vi "GetText.vi"(8 "error in":errorcluster, 11 "EngineTags in":refnum<class "EngineTags.lvclass">) -> (0 "error out":errorcluster, 1 "additional text":string, 2 "text":string, 3 "EngineTags out":refnum<class "EngineTags.lvclass">, 4 "glyph":string)   [LabVIEW 2013, in "PL Framework Configuration Tool.lvlib" / "EngineTags.lvclass"]
uses:
  EngineTags.lvclass
  subVIs/Glyphs Status.ctl
  PL Framework Configuration Tool.lvlib
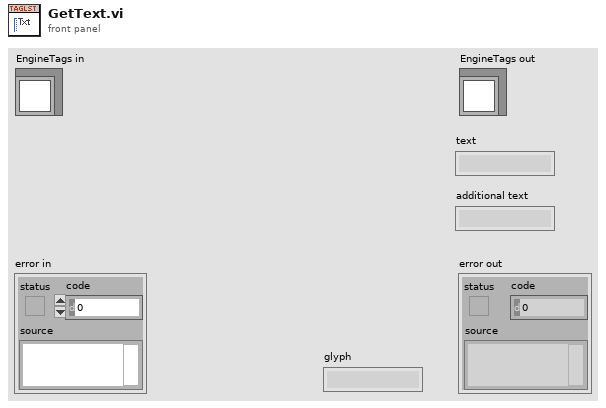
[diagram p1: front panel]
types:
  T1 = typedef "PL Framework Configuration Tool.lvlib/Glyphs Status.ctl" = enum16{"Normal", "Error", "Async"}
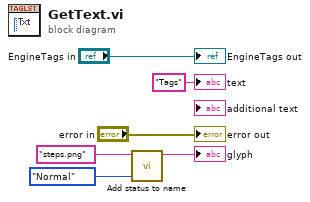
[diagram p0: block diagram]
diagram:
  n1 = call "Add status to name.vi"("Status"=Glyphs_Status."Normal", "Name"="steps.png" ("glyph")) -> ("Name with status"=→"glyph":string)  [unwired: 9 in]
  "error out" <- "error in"
  "EngineTags out" <- "EngineTags in"
  "text" <- "Tags" ("text")
